vi "Voronoi and Delaunay Plot.vi"() -> ()   [LabVIEW 2023]
doc: "The following steps show how to use the Voronoi Diagram VI and Delaunay Triangulation VI.\n\n1) Change <b># of points</b> to set the number of random points that generate.\n2) Run the VI.\n3) Observe the Voronoi diagram, Delaunay triangulation, and the relationship between both of them."
uses:
  <vilib>/Analysis/NI_AAL_Geometry.lvlib
panel:
  out "Voronoi and Delaunay":cluster{dbl[], dbl[]}[](graph)
  in  "# of points":i32=12 min=3 max=10000 step=1
  # "Overview: Demonstrates the use of the Voronoi Diagram and Delaunay Triangulation VIs.\nRequirements: LabVIEW Full Development System\nInstructions: \n1. Change the # of points to set the number of random points that are generated.\n2. Run the VI."
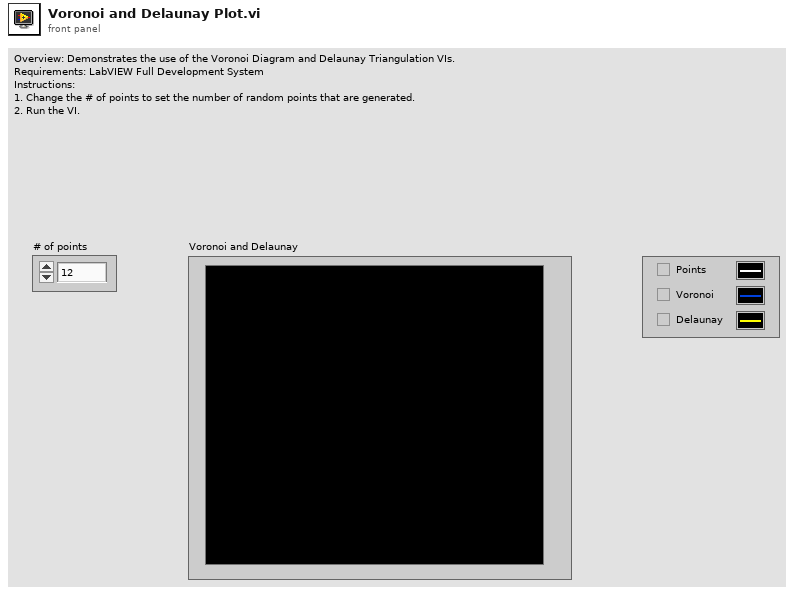
[diagram p1: front panel]
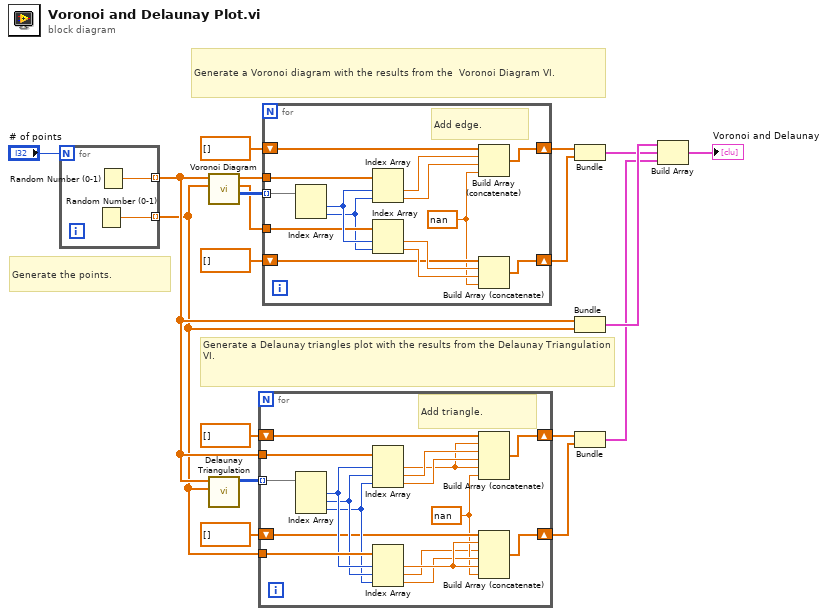
[diagram p0: block diagram]
diagram:
  # "Generate a Voronoi diagram with the results from the  Voronoi Diagram VI."
  # "Generate the points."
  # "Generate a Delaunay triangles plot with the results from the Delaunay Triangulation VI."
  n1 = for {
    N: "# of points" -> [_]
    tunnel: [w21] -> w7 mode=indexing
    tunnel: [w20] -> w6 mode=indexing
    n2 = Random Number (0-1)() -> (number: 0 to 1=w20:dbl)
    n3 = Random Number (0-1)() -> (number: 0 to 1=w21:dbl)
  }
  n4 = call <vilib>:"Voronoi Diagram.vi"("Y"=w6, "X"=w7) -> ("Voronoi Edges"=w19:i32[][], "Voronoi Y"=w13:dbl[], "Voronoi X"=w14:dbl[])  [unwired: 6 in, 1 out]
  n5 = call <vilib>:"Delaunay Triangulation.vi"("Y"=w6, "X"=w7) -> ("Triangles"=w12:i32[][])  [unwired: 8 in, 1 out]
  n6 = for {
    tunnel: w12 -> [w37] mode=indexing
    tunnel: w7 -> [w38]
    tunnel: w6 -> [w33]
    shift-right: [w26] -> w9
    shift-left: dbl[] [] -> [w27]
    shift-right: [w25] -> w8
    shift-left: dbl[] [] -> [w24]
    w23 = nan ("element")
    # "Add triangle."
    n7 = Index Array(array=w37) -> (element #1=w32:i32, element #2=w31:i32, element #3=w30:i32)  [unwired: 3 in]
    n8 = Index Array(array=w38, index #1=w32, index #2=w31, index #3=w30) -> (element #1=w34:dbl, element #2=w36:dbl, element #3=w35:dbl)
    n9 = Index Array(array=w33, index #1=w32, index #2=w31, index #3=w30) -> (element #1=w29:dbl, element #2=w22:dbl, element #3=w28:dbl)
    n10 = Build Array (concatenate)(w27, w34, w36, w35, w34, w23) -> (w26:dbl[])
    n11 = Build Array (concatenate)(w24, w29, w22, w28, w29, w23) -> (w25:dbl[])
  }
  n12 = for {
    tunnel: w19 -> [w52] mode=indexing
    shift-right: [w43] -> w16
    shift-left: dbl[] [] -> [w44]
    shift-right: [w41] -> w15
    shift-left: dbl[] [] -> [w42]
    tunnel: w14 -> [w48]
    tunnel: w13 -> [w47]
    w40 = nan ("element")
    # "Add edge."
    n13 = Index Array(array=w52) -> (element #1=w50:i32, element #2=w39:i32)  [unwired: 2 in]
    n14 = Index Array(array=w48, index #1=w50, index #2=w39) -> (element #1=w46:dbl, element #2=w51:dbl)
    n15 = Index Array(array=w47, index #1=w50, index #2=w39) -> (element #1=w45:dbl, element #2=w49:dbl)
    n16 = Build Array (concatenate)(w44, w46, w51, w40) -> (w43:dbl[])
    n17 = Build Array (concatenate)(w42, w45, w49, w40) -> (w41:dbl[])
  }
  n18 = Bundle(w16, w15) -> (w3:cluster{dbl[], dbl[]})  [unwired: 1 in]
  n19 = Bundle(w7, w6) -> (w4:cluster{dbl[], dbl[]})  [unwired: 1 in]
  n20 = Bundle(w9, w8) -> (w2:cluster{dbl[], dbl[]})  [unwired: 1 in]
  n21 = Build Array(w4, w3, w2) -> (→"Voronoi and Delaunay":cluster{dbl[], dbl[]}[])
